vi "状态自检_v4.vi"(11 "陀螺自检状态字":u8) -> (3 "连接的字符串":string)   [LabVIEW 2012]
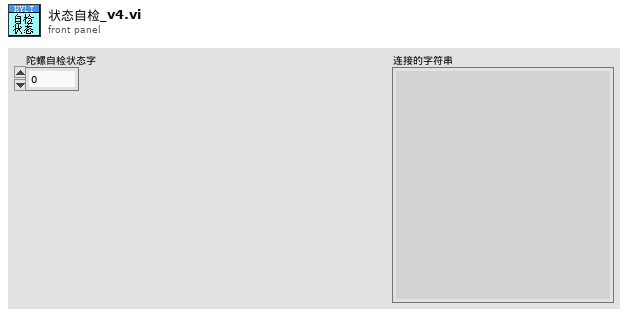
[diagram p1: front panel]
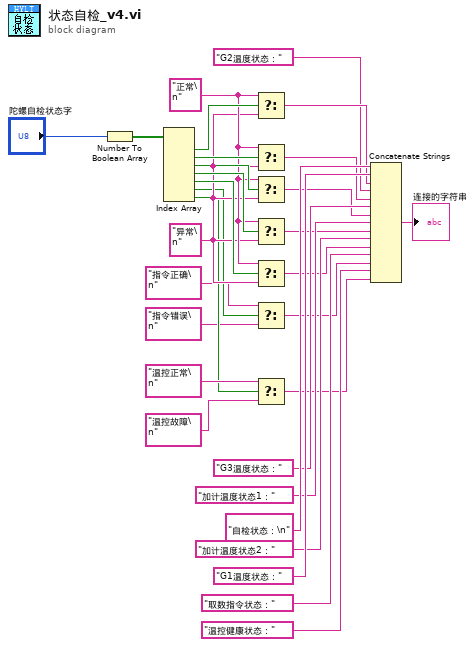
[diagram p0: block diagram]
diagram:
  w13 = "异常\n" ("f")
  w14 = "正常\n" ("主份自检状态及船舱标志")
  n1 = Number To Boolean Array(number="陀螺自检状态字") -> (Boolean array=w29:bool[])
  n2 = Index Array(array=w29) -> (element #1=w28:bool, element #2=w27:bool, element #3=w20:bool, element #4=w17:bool, element #5=w15:bool, element #6=w12:bool, element #7=w4:bool)  [unwired: 7 in]
  n3 = Select(t=w14, s=w28, f=w13) -> (s? t:f=w24:string)
  n4 = Select(t=w14, s=w27, f=w13) -> (s? t:f=w21:string)
  n5 = Select(t=w14, s=w20, f=w13) -> (s? t:f=w19:string)
  n6 = Select(t=w14, s=w17, f=w13) -> (s? t:f=w16:string)
  n7 = Select(t=w14, s=w15, f=w13) -> (s? t:f=w10:string)
  n8 = Select(t="指令正确\n" ("s? t:f"), s=w12, f="指令错误\n" ("s? t:f")) -> (s? t:f=w8:string)
  n9 = Select(t="温控正常\n" ("s? t:f"), s=w4, f="温控故障\n" ("s? t:f")) -> (s? t:f=w3:string)
  n10 = Concatenate Strings("自检状态：\n" ("字符串"), "G1温度状态：" ("s? t:f"), w24, "G2温度状态：" ("s? t:f"), w21, "G3温度状态：" ("s? t:f"), w19, "加计温度状态1：" ("s? t:f"), w16, "加计温度状态2：" ("s? t:f"), w10, "取数指令状态：" ("s? t:f"), w8, "温控健康状态：" ("s? t:f"), w3) -> (→"连接的字符串":string)
